vi "setMEDFilterStatus.vi.vi"(8 "error in (no error)":errorcluster, 9 "MED Filter Active":T1, 10 "Measurement Function (0: Current)":T2, 11 "Electrometer in":refnum<class "Electrometer.lvclass">) -> (0 "error out":errorcluster, 3 "Electrometer out":refnum<class "Electrometer.lvclass">)   [LabVIEW 2016, in "Electrometer.lvclass"]
uses:
  Electrometer.lvclass
  Modes.ctl
  MED Filter Type.ctl
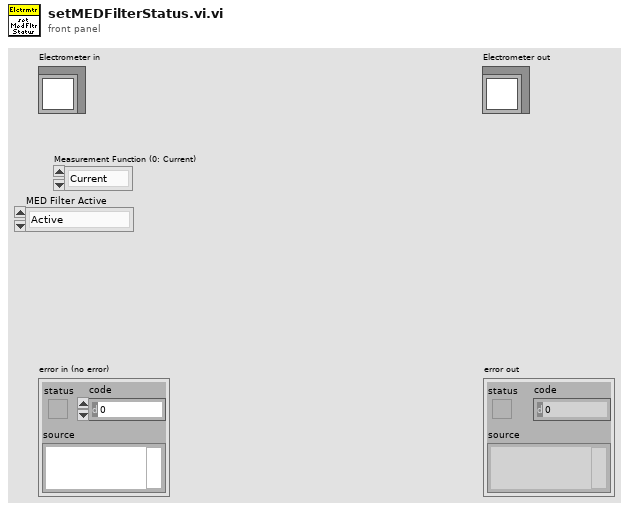
[diagram p1: front panel]
types:
  T1 = typedef "Electrometer.lvclass/MED Filter Type.ctl" = enum16{"Active", "None"}
  T2 = typedef "Electrometer.lvclass/Modes.ctl" = enum16{"Current", "Charge", "Voltage", "Resistance"}
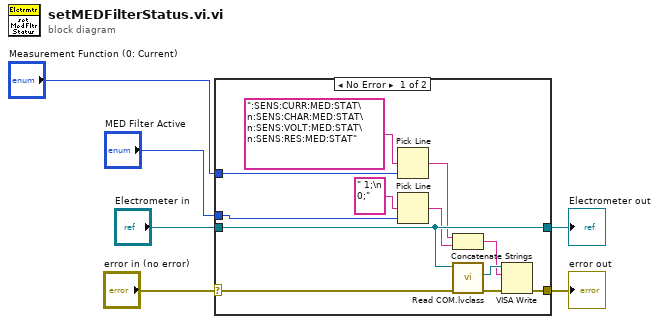
[diagram p0: block diagram]
diagram:
  n1 = case shown="No Error" "error in (no error)" {
    selector: "error in (no error)" -> [w15 w20]
    tunnel: [w12 w20] -> w5
    tunnel: [w14 w19] -> w3
    tunnel: "Electrometer in" -> [w14 w19]
    tunnel: "Measurement Function (0: Current)" -> [w13 _]
    tunnel: "MED Filter Active" -> [w10 _]
    frame No Error {
      n2 = Pick Line(multi-line string=":SENS:CURR:MED:STAT\n:SENS:CHAR:MED:STAT\n:SENS:VOLT:MED:STAT\n:SENS:RES:MED:STAT", line index=w13) -> (output string=w9:string)  [unwired: 1 in]
      n3 = Pick Line(multi-line string=" 1;\n 0;", line index=w10) -> (output string=w8:string)  [unwired: 1 in]
      n4 = Concatenate Strings(w9, w8) -> (w7:string)
      n5 = call "Read COM.lvclass.vi"("error in (no error)"=w15, "Electrometer in"=w14) -> ("error out"=w16:errorcluster, "VISA"=w18:refnum<visa-resource-name>)  [unwired: 7 in, 1 out]
      n6 = VISA Write(VISA resource name=w18, write buffer=w7, error in (no error)=w16) -> (error out=w12:errorcluster)  [unwired: 2 out]
    }
    frame Error {
    }
  }
  "error out" <- w5
  "Electrometer out" <- w3
